vi "Prepare View.vi"(8 "error in":errorcluster, 10 "Cell":refnum<class "Cell.lvclass">, 11 "Cell View Alternating Back Color in":refnum<class "Cell View Alternating Back Color.lvclass">) -> (0 "error out":errorcluster, 3 "Cell View Alternating Back Color out":refnum<class "Cell View Alternating Back Color.lvclass">)   [LabVIEW 2023, in "SourceGrid.lvlib" / "Cell View Alternating Back Color.lvclass"]
uses:
  Cell View Alternating Back Color.lvclass
  Cells/Cell/Cell.lvclass
  Cell View Alternating Back Color.lvclass/Cell View Alternating Back Color.ctl
  D:/git/Sourcegrid-LabVIEW/dll/SourceGrid.dll
  dll/SourceGrid.dll
  Cell View/Cell View.lvclass
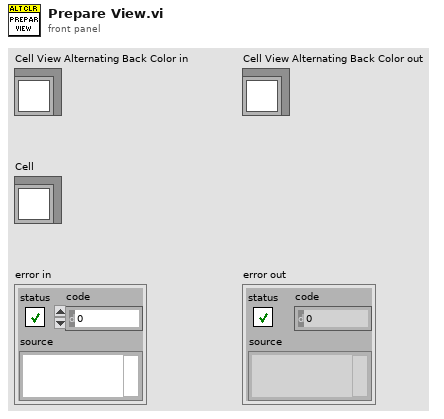
[diagram p1: front panel]
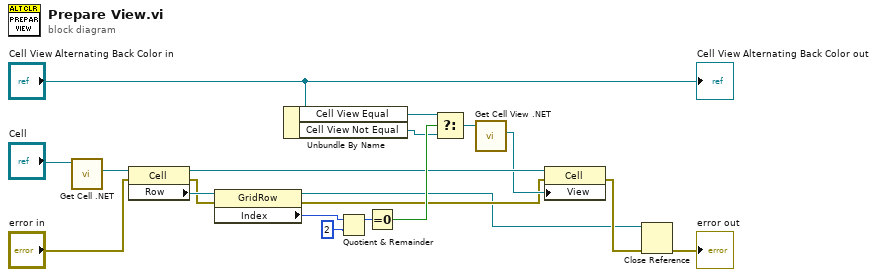
[diagram p0: block diagram]
diagram:
  n1 = call-dynamic "Get Cell .NET.vi"("Cell in"="Cell") -> ("Cell .NET"=w15:refnum<k24>)  [unwired: 9 in, 1 out]
  n2 = property class="Cell"(reference=w15, error in="error in") -> (reference out=w7:refnum<k24>, error out=w13:errorcluster, "Row"=w14:refnum<k24>)
  n3 = property class="GridRow"(reference=w14, error in=w13) -> (reference out=w1:refnum<k24>, error out=w4:errorcluster, "Index"=w11:i32)
  n4 = Unbundle By Name("Cell View Alternating Back Color in") -> ("Cell View Equal"=w9:refnum<class "Cell View.lvclass">, "Cell View Not Equal"=w8:refnum<class "Cell View.lvclass">)
  n5 = Quotient & Remainder(x=w11, y=2) -> (x-y*floor(x/y)=w18:i32)  [unwired: 1 out]
  n6 = Equal To 0?(x=w18) -> (x = 0?=w17:bool)
  n7 = Select(t=w9, s=w17, f=w8) -> (s? t:f=w6:refnum<class "Cell View.lvclass">)
  n8 = call "Get Cell View .NET.vi"("Cell View in"=w6) -> ("Cell View .NET"=w5:refnum<k24>)  [unwired: 9 in, 1 out]
  n9 = property class="Cell"(reference=w7, error in=w4, "View"=w5) -> (error out=w3:errorcluster)  [unwired: 1 out]
  n10 = Close Reference(reference=w1, error in (no error)=w3) -> (error out=→"error out":errorcluster)
  "Cell View Alternating Back Color out" <- "Cell View Alternating Back Color in"
